vi "Untitled 1.vi"() -> ()   [LabVIEW 2024]
panel:
  out "Speed(ms)":dbl
  in  "Set Temp":dbl(slide) scale=0.0..10.0
  out "Temp, C":dbl(slide) scale=0.0..100.0
  out "Vmj, V":dbl
  out "Vdiff, V":dbl
  in  "stop":bool
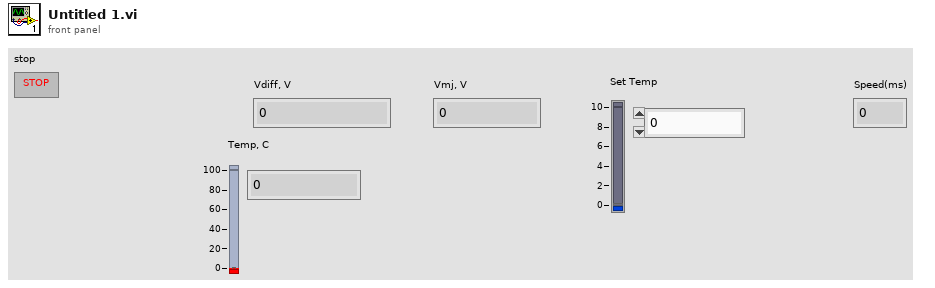
[diagram p1: front panel]
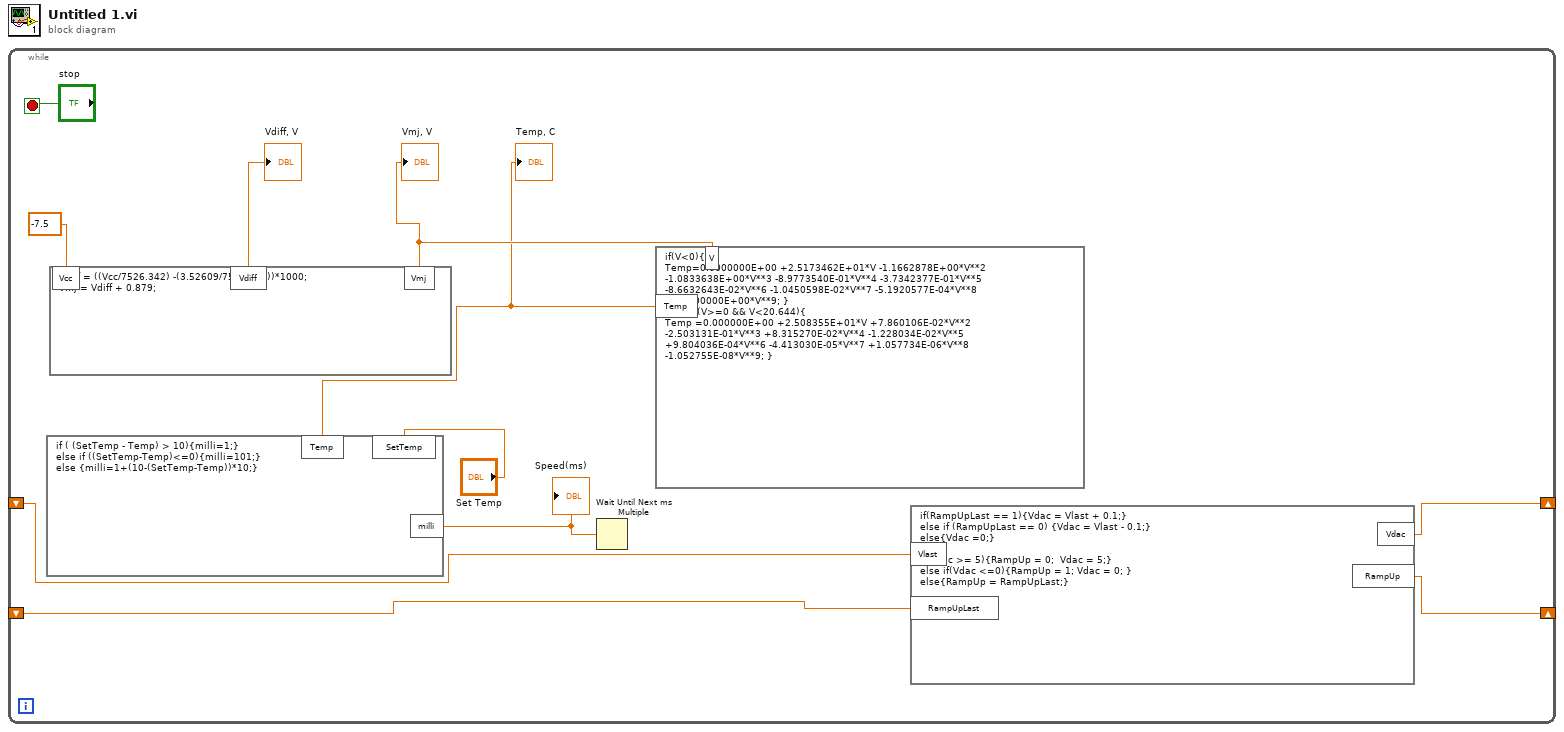
[diagram p0: block diagram]
diagram:
  n1 = while {
    shift-right: [w10] -> _
    shift-left: _ -> [w9]
    shift-right: [w7] -> _
    shift-left: _ -> [w8]
    stop <- "stop" stop-if-true
    n2 = formula code="Vdiff = ((Vcc/7526.342) -(3.52609/7526.342))*1000;\nVmj = Vdiff + 0.879;"("Vcc"=-7.5) -> ("Vdiff"=→"Vdiff, V":dbl, "Vmj"=w3:dbl)
    "Vmj, V" <- w3
    n3 = formula code="if(V<0){\nTemp=0.0000000E+00 +2.5173462E+01*V -1.1662878E+00*V**2\n-1.0833638E+00*V**3 -8.9773540E-01*V**4 -3.7342377E-01*V**5\n-8.6632643E-02*V**6 -1.0450598E-02*V**7 -5.1920577E-04*V**8\n+0.0000000E+00*V**9; }\nelse if (V>=0 && V<20.644){\nTemp =0.000000E+00 +2.508355E+01*V +7.860106E-02*V**2 \n-2.503131E-01*V**3 +8.315270E-02*V**4 -1.228034E-02*V**5 \n+9.804036E-04*V**6 -4.413030E-05*V**7 +1.057734E-06*V**8 \n-1.052755E-08*V**9; }"("V"=w3) -> ("Temp"=w1:dbl)
    "Temp, C" <- w1
    n4 = formula code="if ( (SetTemp - Temp) > 10){milli=1;}\nelse if ((SetTemp-Temp)<=0){milli=101;}\nelse {milli=1+(10-(SetTemp-Temp))*10;}"("SetTemp"="Set Temp", "Temp"=w1) -> ("milli"=w5:dbl)
    "Speed(ms)" <- w5
    n5 = Wait Until Next ms Multiple(millisecond multiple=w5) -> ()  [unwired: 1 out]
    n6 = formula code="if(RampUpLast == 1){Vdac = Vlast + 0.1;}\nelse if (RampUpLast == 0) {Vdac = Vlast - 0.1;}\nelse{Vdac =0;}\n\nif(Vdac >= 5){RampUp = 0;  Vdac = 5;}\nelse if(Vdac <=0){RampUp = 1; Vdac = 0; }\nelse{RampUp = RampUpLast;}"("Vlast"=w9, "RampUpLast"=w8) -> ("Vdac"=w10:dbl, "RampUp"=w7:dbl)
  }
